vi "DAQ-node.vi"() -> ()   [LabVIEW 2024]
uses:
  DAQ-node_streamIO_settings.ctl
  <vilib>/DAQmx/read.llb/DAQmx Read (Analog 2D DBL NChan NSamp).vi
  <vilib>/DAQmx/create/channels.llb/DAQmx Create Channel (AI-Voltage-Basic).vi
  <vilib>/DAQmx/configure/timing.llb/DAQmx Timing (Sample Clock).vi
  <vilib>/DAQmx/miscellaneous.llb/DAQmx Fill In Error Info.vi
panel:
  in  "Reader Endpoint":string="CTR001"
  in  "Writer Endpoint":string="DAQ001"
  in  "Reader IP Addr":string="localhost"
  out "Waveform Chart":dbl[][](graph)
  in  "stop":bool
  in  "error in":errorcluster
  out "error out":errorcluster
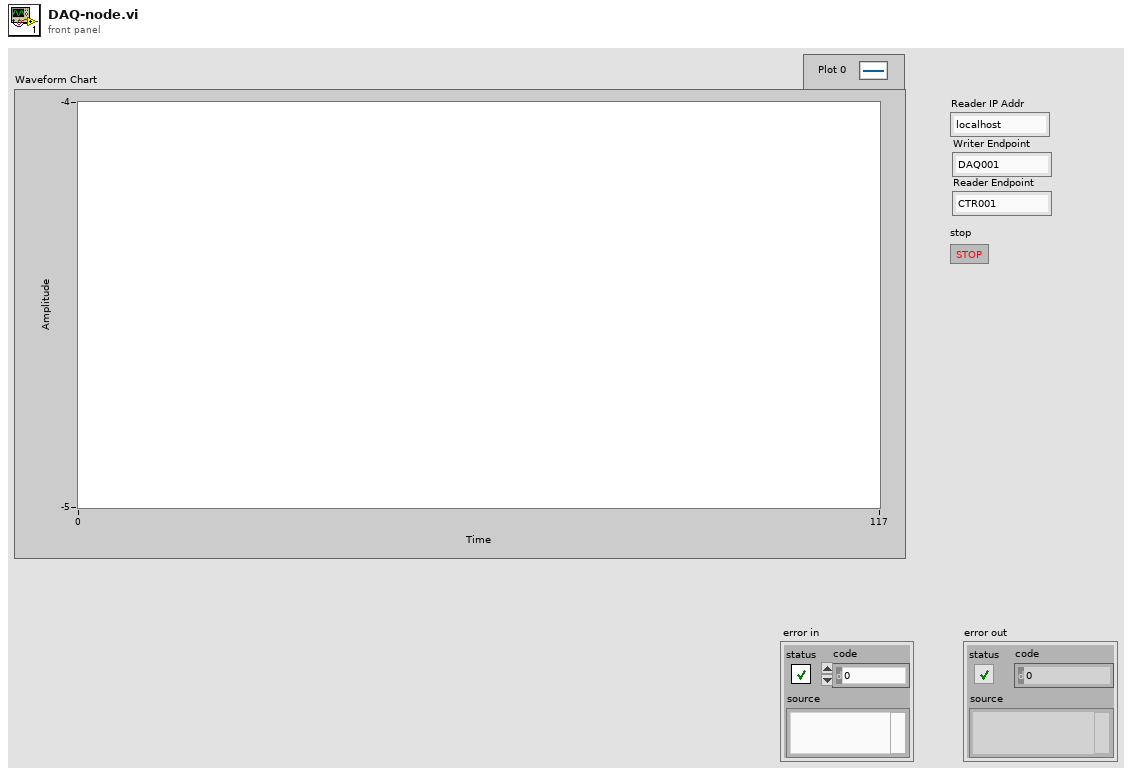
[diagram p1: front panel]
types:
  T1 = typedef "DAQ-node_streamIO_settings.ctl" = cluster{"Reader IP Addr":string, "Writer Endpoint":string, "Reader Endpoint":string, "Channel Definitions":cluster{"refdes":string, "channel":string, "offset":dbl, "slope":dbl, "units":string}[], "Writer Endpoint Ref":refnum<k21>, "Reader Endpoint Ref":refnum<k21>, "steam error":errorcluster}
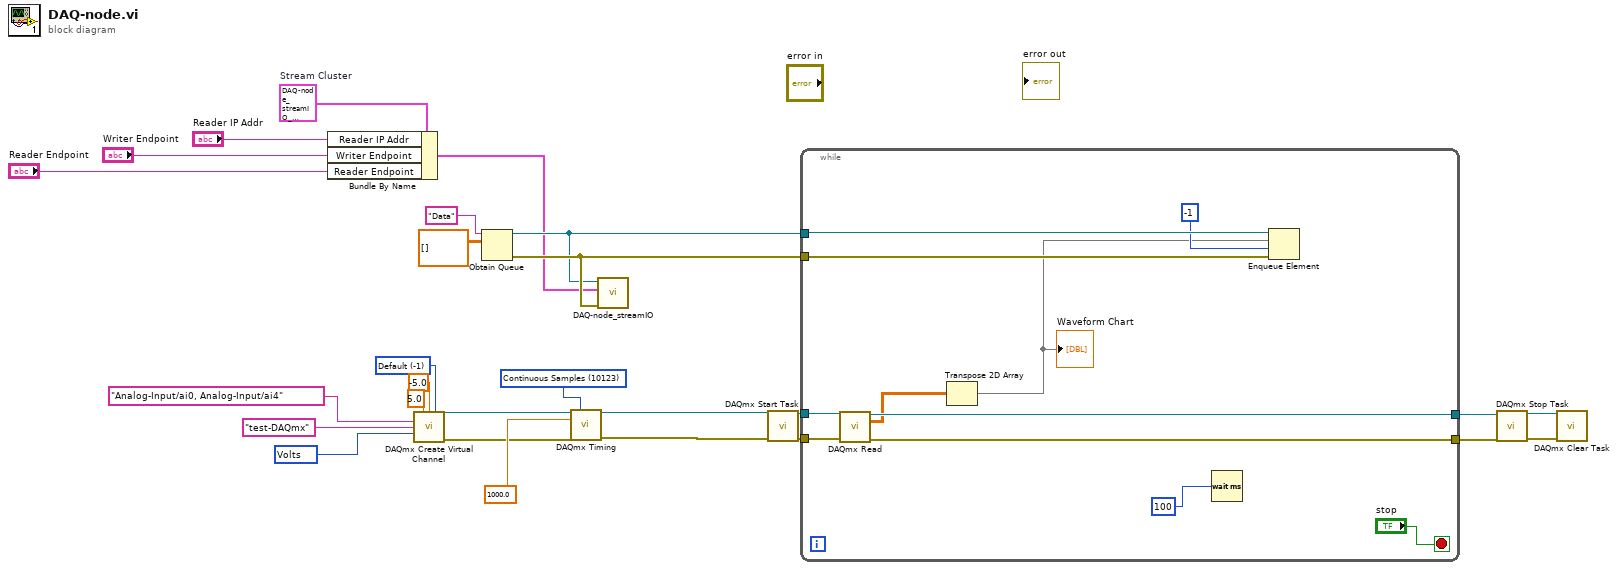
[diagram p0: block diagram]
diagram:
  w4 = T1 {"Reader IP Addr"="localhost", "Writer Endpoint"="DAQ001", "Reader Endpoint"="CTR001", "Channel Definitions"=[], "Writer Endpoint Ref"="", "Reader Endpoint Ref"="", "steam error"={"status"=FALSE, "code"=0, "source"=""}}  # Stream Cluster
  w17 = 10123 items=["Finite Samples"=10178, "Continuous Samples"=10123, "Hardware Timed Single Point"=12522] ("sample mode")
  w20 = 10348 items=["Volts"=10348, "From Custom Scale"=10065] ("units")
  w25 = -1 items=["Default"=-1, "RSE"=10083, "NRSE"=10078, "Differential"=10106, "Pseudodifferential"=12529] ("input terminal configuration")
  n1 = Bundle By Name(cluster=w4, "Reader IP Addr"="Reader IP Addr", "Writer Endpoint"="Writer Endpoint", "Reader Endpoint"="Reader Endpoint") -> (w7:T1)
  n2 = call-poly <vilib>:"DAQmx Create Virtual Channel.vi"("maximum value"=5.0, "minimum value"=-5.0, "input terminal configuration"=w25, "physical channels"=tag "Analog-Input/ai0, Analog-Input/ai4", "name to assign"="test-DAQmx", "units"=w20) -> ("task out"=w16:refnum<k21>, "error out"=w10:errorcluster)  [unwired: 8 in]
  n3 = Obtain Queue(name (unnamed)="Data", element data type=dbl[][] [] ("data")) -> (queue out=w8:refnum<queue>, error out=w9:errorcluster)  [unwired: 3 in, 1 out]
  n4 = call-poly <vilib>:"DAQmx Timing.vi"("task/channels in"=w16, "sample mode"=w17, "rate"=1000.0, "error in"=w10) -> ("task out"=w18:refnum<k21>, "error out"=w19:errorcluster)  [unwired: 10 in]
  n5 = call "DAQ-node_streamIO.vi"("error in"=w9, "Stream Cluster"=w7, "queue out"=w8) -> ()  [unwired: 7 in, 2 out]
  n6 = call <vilib>:"DAQmx Start Task.vi"("task/channels in"=w18, "error in"=w19) -> ("task out"=w14:refnum<k21>, "error out"=w13:errorcluster)  [unwired: 12 in]
  n7 = while {
    tunnel: w14 -> [w37]
    tunnel: w13 -> [w36]
    tunnel: [w35] -> w12
    tunnel: [w34] -> w11
    tunnel: w8 -> [w33]
    tunnel: w9 -> [w32]
    stop <- "stop" stop-if-true
    n8 = call-poly <vilib>:"DAQmx Read.vi"("task/channels in"=w37, "error in"=w36) -> ("task out"=w34:refnum<k21>, "data"=w29:dbl[][], "error out"=w35:errorcluster)  [unwired: 11 in]
    n9 = Transpose 2D Array(2D array=w29) -> (transposed array=w28:dbl[][])
    "Waveform Chart" <- w28
    n10 = Wait (ms)(milliseconds to wait=u32 100) -> ()  [unwired: 1 out]
    n11 = Enqueue Element(queue=w33, element=w28, timeout in ms (-1)=-1, error in (no error)=w32) -> ()  [unwired: 3 out]
  }
  n12 = call <vilib>:"DAQmx Stop Task.vi"("task/channels in"=w11, "error in"=w12) -> ("task out"=w27:refnum<k21>, "error out"=w26:errorcluster)  [unwired: 12 in]
  n13 = call <vilib>:"DAQmx Clear Task.vi"("task in"=w27, "error in"=w26) -> ()  [unwired: 13 in, 1 out]
